vi "Autonomous Independent.vi"   [LabVIEW 2017]
doc: "This VI is called when autonomous begins, and will automatically be terminated when autonomous ends. You can carry out timed or sensor driven robot movement independently without needing to return to the caller."
uses:
  Control 1.ctl
  <vilib>/Rock Robotics/Network Tables/NT Read String.vi
  <vilib>/Rock Robotics/WPI/Utilities/WPI_GetSetVariantRefNum.vi
panel:
  # "Be sure to right-click and choose Data Operations>>Make Current Value default if you want to save the array values with the VI"
types:
  T1 = typedef "Control 1.ctl" = enum16{"AndarFrente", "Zerador", "DobraDireita", "Zerador1", "VoltarDireita", "Zerador2", "AndarRe", "Fatality", "AndarDireita", "Zerador3", "DobrarDireita2", "Zeador4", "Parar", "Parar2", "Zerador5", "Zerador6", "Zerador7", "Parar3"}
  T2 = typedef "WPI_MotorControlDeviceRef.ctl" = cluster{"DeviceStatus":errorcluster, "Type":T3, "PWM":cluster{"PWM Channel":T4, "DeadBand":T5}, "CAN":cluster{"Device Number":u8, "SetOutput VI Ref":variant, "GetOutput VI Ref":variant, "Enable VI Ref":variant, "Disable VI Ref":variant, "Data":variant}, "Invert":bool, "DIO PWM":cluster{"PWM \"Enable\" Channel":T4, "DIOChannel":T6, "PWM Rate":dbl}}
  T3 = typedef "WPI_MotorControlType.ctl" = enum16{"PWM", "CAN", "DIO PWM"}
  T4 = typedef "FPGA_DIOPWMChannel.ctl" = enum8{"PWM 0", "PWM 1", "PWM 2", "PWM 3", "PWM 4", "PWM 5", "PWM 6", "PWM 7", "PWM 8", "PWM 9", "PWM MXP 0", "PWM MXP 1", "PWM MXP 2", "PWM MXP 3", "PWM MXP 4", "PWM MXP 5", "PWM MXP 6", "PWM MXP 7", "PWM MXP 8", "PWM MXP 9", "Invalid"}
  T5 = typedef "WPI_PWMDeadband.ctl" = cluster{"Name":string, "maxPositivePwm":i32, "minPositivePwm":i32, "centerPwm":i32, "maxNegativePwm":i32, "minNegativePwm":i32, "angularRange":u16}
  T6 = typedef "FPGA_DIOChannel.ctl" = enum8{"DIO 0", "DIO 1", "DIO 2", "DIO 3", "DIO 4", "DIO 5", "DIO 6", "DIO 7", "DIO 8", "DIO 9", "DIO MXP 0", "DIO MXP 1", "DIO MXP 2", "DIO MXP 3", "DIO MXP 4", "DIO MXP 5", "DIO MXP 6", "DIO MXP 7", "DIO MXP 8", "DIO MXP 9", "DIO MXP 10", "DIO MXP 11", "DIO MXP 12", "DIO MXP 13", "DIO MXP 14", "DIO MXP 15", "SPI Port CS1", "SPI Port CS2", "SPI Port CS3", "SPI Port MISO", "SPI Port MOSI", "Invalid"}
  T7 = typedef "WPI_RobotDriveDevRef.ctl" = cluster{"DevStatus":errorcluster, "Motors[]":T2[], "Square Inputs":bool, "Max Output":dbl}
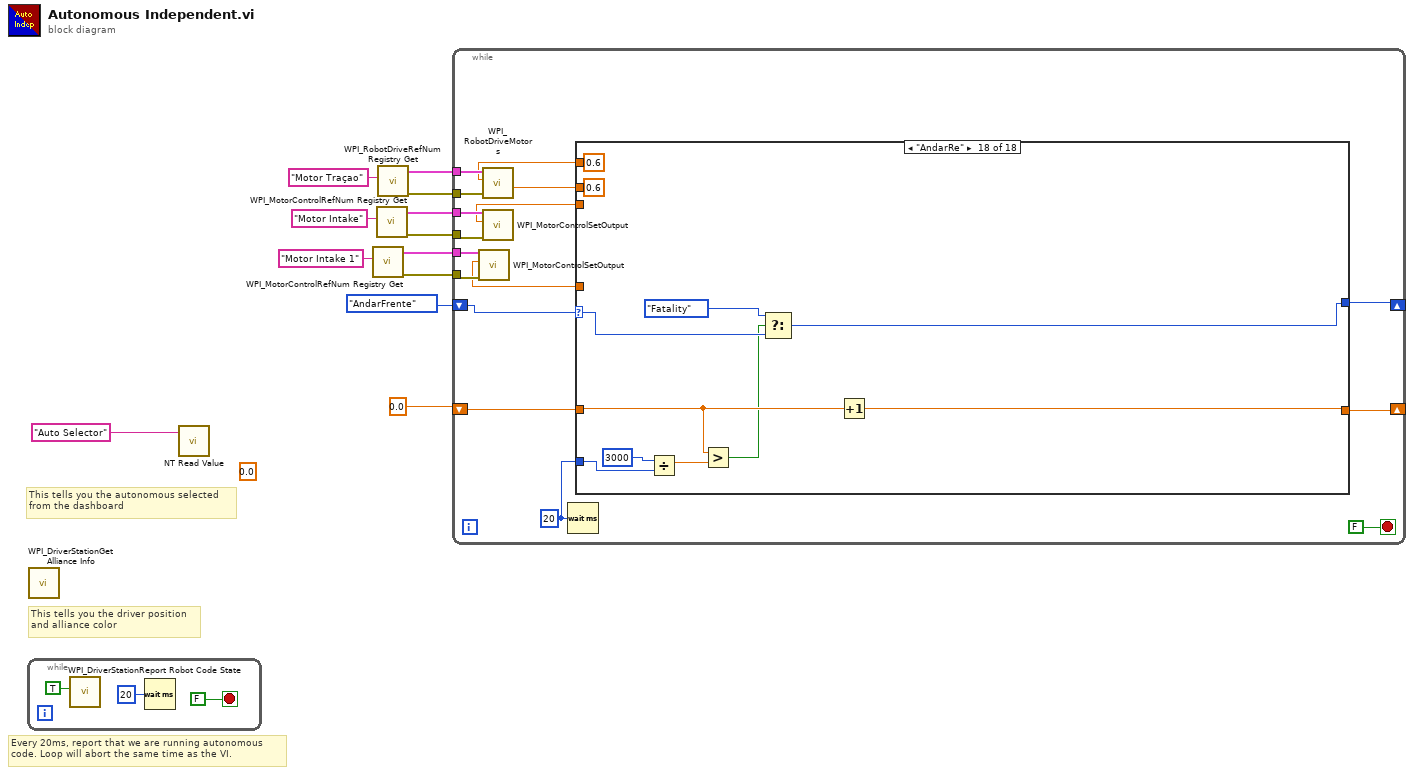
[diagram p0: block diagram]
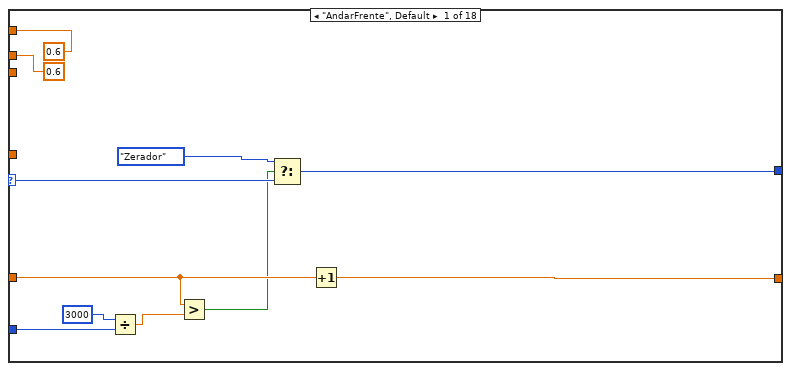
[diagram p2: hidden frame]
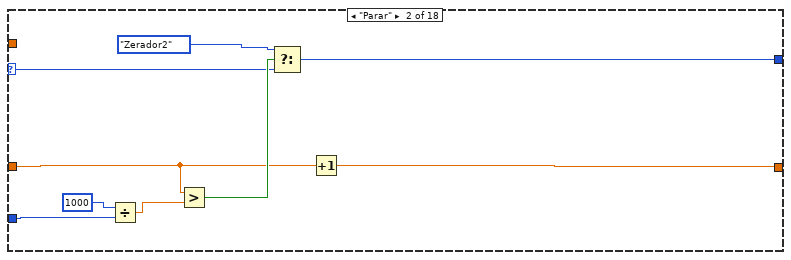
[diagram p3: hidden frame]
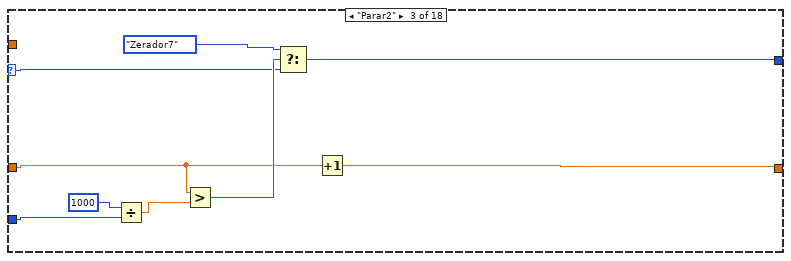
[diagram p4: hidden frame]
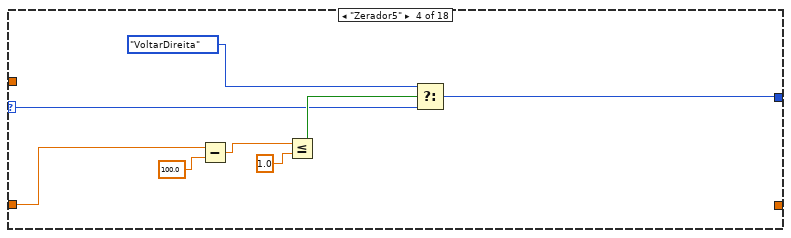
[diagram p5: hidden frame]
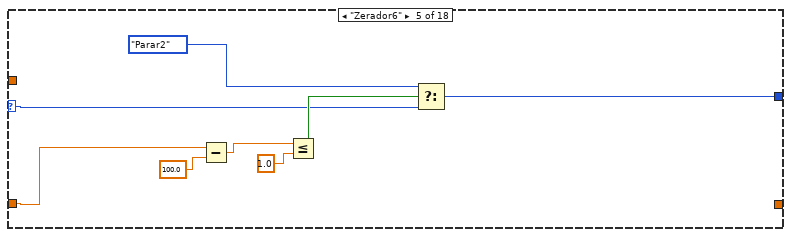
[diagram p6: hidden frame]
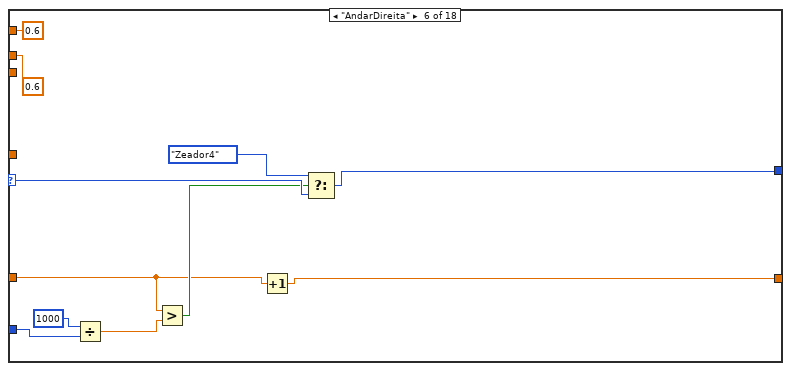
[diagram p7: hidden frame]
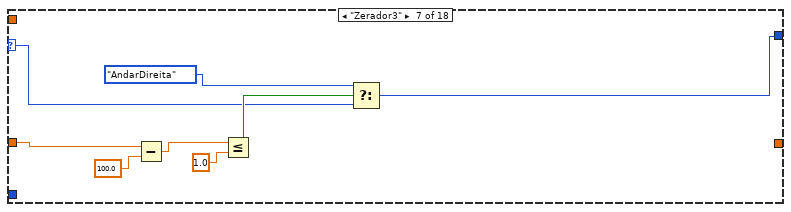
[diagram p8: hidden frame]
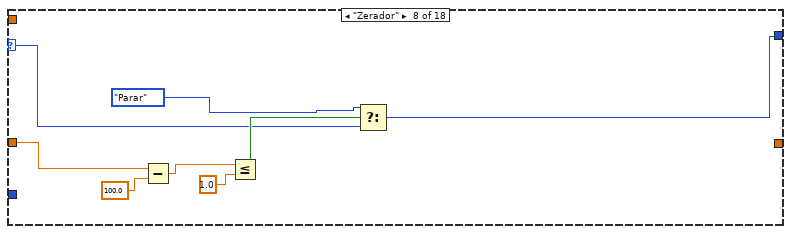
[diagram p9: hidden frame]
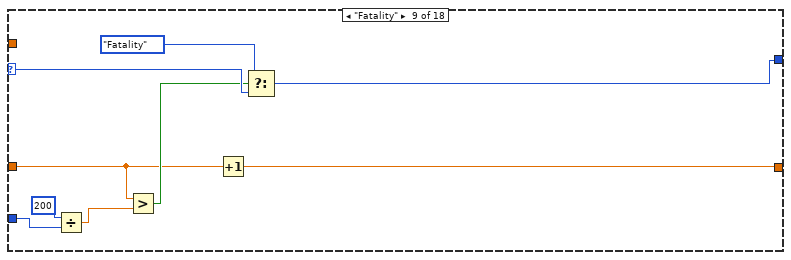
[diagram p10: hidden frame]
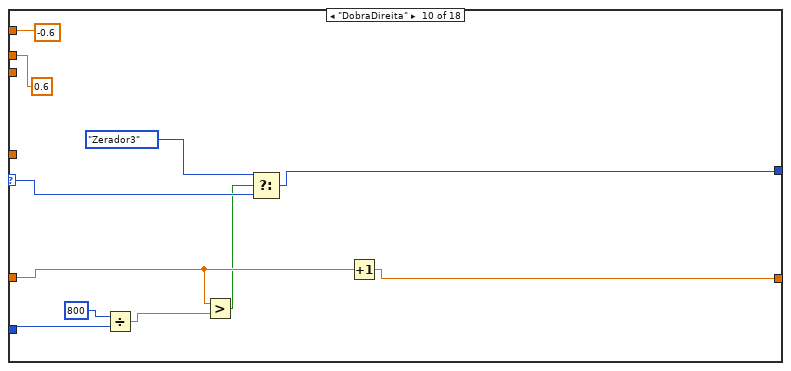
[diagram p11: hidden frame]
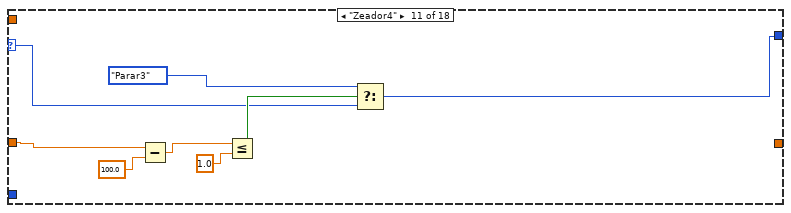
[diagram p12: hidden frame]
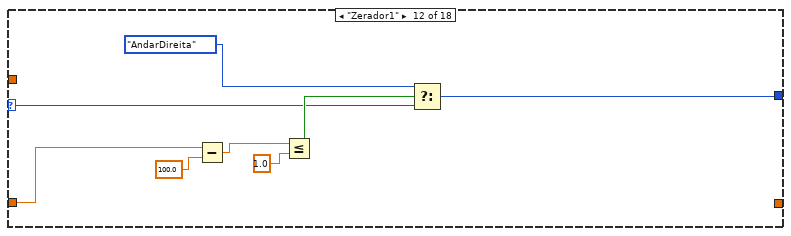
[diagram p13: hidden frame]
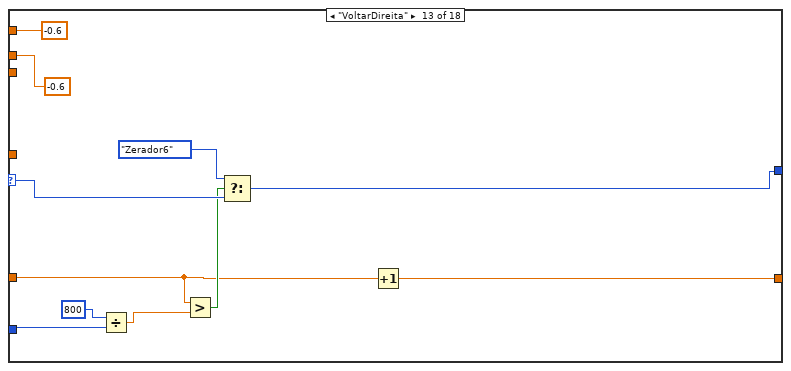
[diagram p14: hidden frame]
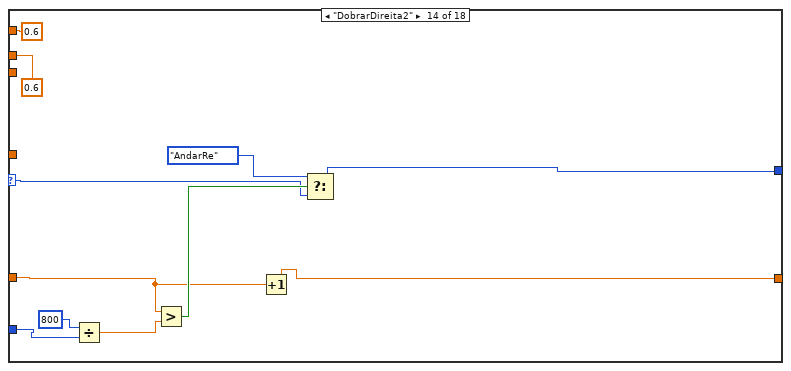
[diagram p15: hidden frame]
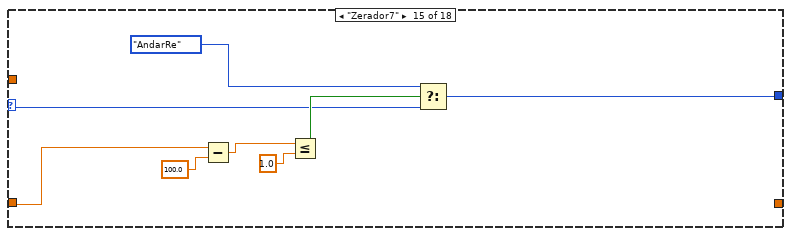
[diagram p16: hidden frame]
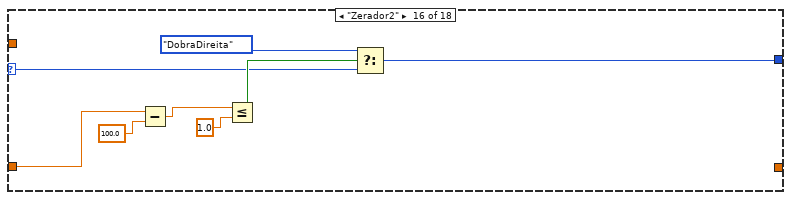
[diagram p17: hidden frame]
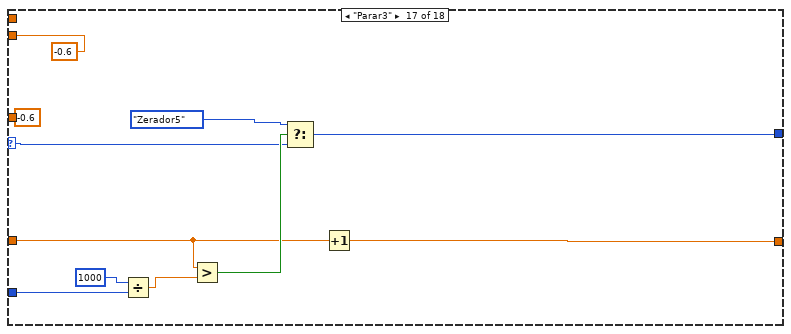
[diagram p18: hidden frame]
diagram:
  (unwired) 0.0
  # "This tells you the autonomous selected\nfrom the dashboard"
  # "Every 20ms, report that we are running autonomous\ncode. Loop will abort the same time as the VI."
  # "This tells you the driver position\nand alliance color"
  n1 = while {
    stop <- FALSE stop-if-true
    n2 = call <vilib>:"WPI_DriverStationReport Robot Code State.vi"("Autonomous"=TRUE) -> ()  [unwired: 10 in, 1 out]
    n3 = Wait (ms)(milliseconds to wait=u32 20) -> ()  [unwired: 1 out]
  }
  n4 = call <vilib>:"WPI_DriverStationGet Alliance Info.vi"() -> ()  [unwired: 12 out]
  n5 = call-poly <vilib>:"NT Read Value.vi"("Name"="Auto Selector") -> ()  [unwired: 9 in, 2 out]
  n6 = call <vilib>:"WPI_MotorControlRefNum Registry Get.vi"("refnum name"="Motor Intake 1") -> ("error out"=w2:errorcluster, "MotorControlDevRef"=w1:T2)  [unwired: 9 in]
  n7 = call <vilib>:"WPI_MotorControlRefNum Registry Get.vi"("refnum name"="Motor Intake") -> ("error out"=w5:errorcluster, "MotorControlDevRef"=w6:T2)  [unwired: 9 in]
  n8 = call <vilib>:"WPI_RobotDriveRefNum Registry Get.vi"("refnum name"="Motor Traçao") -> ("error out"=w8:errorcluster, "RobotDriveDevRef"=w9:T7)  [unwired: 9 in]
  n9 = while {
    shift-right: [w24] -> _
    shift-left: Control_1."AndarFrente" -> [w31]
    shift-right: [w29] -> _
    shift-left: 0.0 -> [w30]
    tunnel: w9 -> [w28]
    tunnel: w8 -> [w27]
    tunnel: w6 -> [w21]
    tunnel: w5 -> [w20]
    tunnel: w1 -> [w19]
    tunnel: w2 -> [w18]
    stop <- FALSE stop-if-true
    w25 = u32 20 ("milliseconds to wait")
    n10 = Wait (ms)(milliseconds to wait=w25) -> ()  [unwired: 1 out]
    n11 = case shown="\"AndarRe\"" w31 {
      selector: w31 -> [w42 w43 w56 w62 w70 w86 w89 w98 w112 w121 w126 w134 w150 w155 w163 w172 w182 w198]
      tunnel: [w41 w44 w52 w61 w69 w85 w88 w97 w104 w114 w124 w135 w141 w151 w162 w173 w181 w197] -> w24
      tunnel: w30 -> [w37 w46 w55 w63 w71 w82 w90 w103 w106 w118 w125 w133 w147 w153 w164 w171 w184 w192]
      tunnel: [w40 w45 w53 _ _ w84 _ _ w110 w120 _ _ w149 w152 _ _ w180 w196] -> w29
      tunnel: [0.6 ("LeftSpeed") _ _ _ _ 0.6 ("LeftSpeed") _ _ _ -0.6 ("LeftSpeed") _ _ -0.6 ("LeftSpeed") 0.6 ("LeftSpeed") _ _ _ 0.6 ("LeftSpeed")] -> w26
      tunnel: [0.6 ("RightSpeed") _ _ _ _ 0.6 ("RightSpeed") _ _ _ 0.6 ("RightSpeed") _ _ -0.6 ("RightSpeed") 0.6 ("RightSpeed") _ _ _ 0.6 ("RightSpeed")] -> w22
      tunnel: w25 -> [w35 w47 w54 _ _ w80 _ _ w109 w117 _ _ w145 w154 _ _ w183 w195]
      tunnel: [_ _ _ _ _ _ _ _ _ _ _ _ _ _ _ _ -0.6 ("RightSpeed") _] -> w17
      tunnel: [_ _ _ _ _ _ _ _ _ _ _ _ _ _ _ _ -0.6 ("Output") _] -> w16
      frame "AndarFrente", Default {
        n12 = Divide(x=u32 3000, y=w35) -> (x/y=w36:dbl)
        n13 = Greater?(x=w37, y=w36) -> (0:w33:bool)
        n14 = Select(t=Control_1."Zerador" ("Enum"), s=w33, f=w42) -> (s? t:f=w41:T1)
        n15 = Increment(x=w37) -> (x+1=w40:dbl)
      }
      frame "Parar" {
        n16 = Divide(x=u32 1000, y=w47) -> (x/y=w51:dbl)
        n17 = Greater?(x=w46, y=w51) -> (0:w49:bool)
        n18 = Select(t=Control_1."Zerador2" ("Enum"), s=w49, f=w43) -> (s? t:f=w44:T1)
        n19 = Increment(x=w46) -> (x+1=w45:dbl)
      }
      frame "Parar2" {
        n20 = Divide(x=u32 1000, y=w54) -> (x/y=w60:dbl)
        n21 = Greater?(x=w55, y=w60) -> (0:w58:bool)
        n22 = Select(t=Control_1."Zerador7" ("Enum"), s=w58, f=w56) -> (s? t:f=w52:T1)
        n23 = Increment(x=w55) -> (x+1=w53:dbl)
      }
      frame "Zerador5" {
        n24 = Subtract(x=w63, y=100.0) -> (x-y=w67:dbl)
        n25 = Less Or Equal?(x=w67, y=1.0) -> (x <= y?=w65:bool)
        n26 = Select(t=Control_1."VoltarDireita" ("Enum"), s=w65, f=w62) -> (s? t:f=w61:T1)
      }
      frame "Zerador6" {
        n27 = Subtract(x=w71, y=100.0) -> (x-y=w75:dbl)
        n28 = Less Or Equal?(x=w75, y=1.0) -> (x <= y?=w73:bool)
        n29 = Select(t=Control_1."Parar2" ("Enum"), s=w73, f=w70) -> (s? t:f=w69:T1)
      }
      frame "AndarDireita" {
        n30 = Divide(x=u32 1000, y=w80) -> (x/y=w81:dbl)
        n31 = Greater?(x=w82, y=w81) -> (0:w83:bool)
        n32 = Increment(x=w82) -> (x+1=w84:dbl)
        n33 = Select(t=Control_1."Zeador4", s=w83, f=w86) -> (s? t:f=w85:T1)
      }
      frame "Zerador3" {
        n34 = Subtract(x=w90, y=100.0) -> (x-y=w94:dbl)
        n35 = Less Or Equal?(x=w94, y=1.0) -> (x <= y?=w95:bool)
        n36 = Select(t=Control_1."AndarDireita" ("Enum"), s=w95, f=w89) -> (s? t:f=w88:T1)
      }
      frame "Zerador" {
        n37 = Subtract(x=w103, y=100.0) -> (x-y=w101:dbl)
        n38 = Less Or Equal?(x=w101, y=1.0) -> (x <= y?=w99:bool)
        n39 = Select(t=Control_1."Parar" ("Enum"), s=w99, f=w98) -> (s? t:f=w97:T1)
      }
      frame "Fatality" {
        n40 = Divide(x=u32 200, y=w109) -> (x/y=w108:dbl)
        n41 = Greater?(x=w106, y=w108) -> (0:w107:bool)
        n42 = Increment(x=w106) -> (x+1=w110:dbl)
        n43 = Select(t=Control_1."Fatality" ("Enum"), s=w107, f=w112) -> (s? t:f=w104:T1)
      }
      frame "DobraDireita" {
        n44 = Divide(x=u32 800, y=w117) -> (x/y=w119:dbl)
        n45 = Greater?(x=w118, y=w119) -> (0:w115:bool)
        n46 = Select(t=Control_1."Zerador3" ("Enum"), s=w115, f=w121) -> (s? t:f=w114:T1)
        n47 = Increment(x=w118) -> (x+1=w120:dbl)
      }
      frame "Zeador4" {
        n48 = Subtract(x=w125, y=100.0) -> (x-y=w130:dbl)
        n49 = Less Or Equal?(x=w130, y=1.0) -> (x <= y?=w131:bool)
        n50 = Select(t=Control_1."Parar3" ("Enum"), s=w131, f=w126) -> (s? t:f=w124:T1)
      }
      frame "Zerador1" {
        n51 = Subtract(x=w133, y=100.0) -> (x-y=w138:dbl)
        n52 = Less Or Equal?(x=w138, y=1.0) -> (x <= y?=w136:bool)
        n53 = Select(t=Control_1."AndarDireita" ("Enum"), s=w136, f=w134) -> (s? t:f=w135:T1)
      }
      frame "VoltarDireita" {
        n54 = Divide(x=u32 800, y=w145) -> (x/y=w146:dbl)
        n55 = Greater?(x=w147, y=w146) -> (0:w148:bool)
        n56 = Select(t=Control_1."Zerador6" ("Enum"), s=w148, f=w150) -> (s? t:f=w141:T1)
        n57 = Increment(x=w147) -> (x+1=w149:dbl)
      }
      frame "DobrarDireita2" {
        n58 = Divide(x=u32 800, y=w154) -> (x/y=w161:dbl)
        n59 = Greater?(x=w153, y=w161) -> (0:w160:bool)
        n60 = Increment(x=w153) -> (x+1=w152:dbl)
        n61 = Select(t=Control_1."AndarRe", s=w160, f=w155) -> (s? t:f=w151:T1)
      }
      frame "Zerador7" {
        n62 = Subtract(x=w164, y=100.0) -> (x-y=w168:dbl)
        n63 = Less Or Equal?(x=w168, y=1.0) -> (x <= y?=w169:bool)
        n64 = Select(t=Control_1."AndarRe" ("Enum"), s=w169, f=w163) -> (s? t:f=w162:T1)
      }
      frame "Zerador2" {
        n65 = Subtract(x=w171, y=100.0) -> (x-y=w176:dbl)
        n66 = Less Or Equal?(x=w176, y=1.0) -> (x <= y?=w177:bool)
        n67 = Select(t=Control_1."DobraDireita" ("Enum"), s=w177, f=w172) -> (s? t:f=w173:T1)
      }
      frame "Parar3" {
        n68 = Divide(x=u32 1000, y=w183) -> (x/y=w188:dbl)
        n69 = Greater?(x=w184, y=w188) -> (0:w186:bool)
        n70 = Select(t=Control_1."Zerador5" ("Enum"), s=w186, f=w182) -> (s? t:f=w181:T1)
        n71 = Increment(x=w184) -> (x+1=w180:dbl)
      }
      frame "AndarRe" {
        n72 = Divide(x=u32 3000, y=w195) -> (x/y=w193:dbl)
        n73 = Greater?(x=w192, y=w193) -> (0:w191:bool)
        n74 = Select(t=Control_1."Fatality" ("Enum"), s=w191, f=w198) -> (s? t:f=w197:T1)
        n75 = Increment(x=w192) -> (x+1=w196:dbl)
      }
    }
    n76 = call <vilib>:"WPI_MotorControlSetOutput.vi"("error in (no error)"=w18, "Output"=w16, "MotorControlDevRef"=w19) -> ()  [unwired: 6 in, 3 out]
    n77 = call <vilib>:"WPI_RobotDriveMotors.vi"("error in (no error)"=w27, "RightSpeed"=w22, "LeftSpeed"=w26, "RobotDriveDevRef"=w28) -> ()  [unwired: 5 in, 3 out]
    n78 = call <vilib>:"WPI_MotorControlSetOutput.vi"("error in (no error)"=w20, "Output"=w17, "MotorControlDevRef"=w21) -> ()  [unwired: 6 in, 3 out]
  }
